vi "Get Selected Device info.vi"(0 "Boolean":bool, 5 "Selected Device":string, 9 "Virtual Devices Core Info":string[][](array[string]), 11 "error in (no error)":errorcluster) -> (4 "Virtual Device Variable List":string[](array[string]), 6 "Actual Device List":string[](array[string]), 8 ">Device Variables (Settable): Default val, Min, Max etc >":string[][](array[string]), 10 ">Selected Device>":string, 15 "error out":errorcluster)   [LabVIEW 2020]
uses:
  Shared/MySQL/Preset Query Enum.ctl
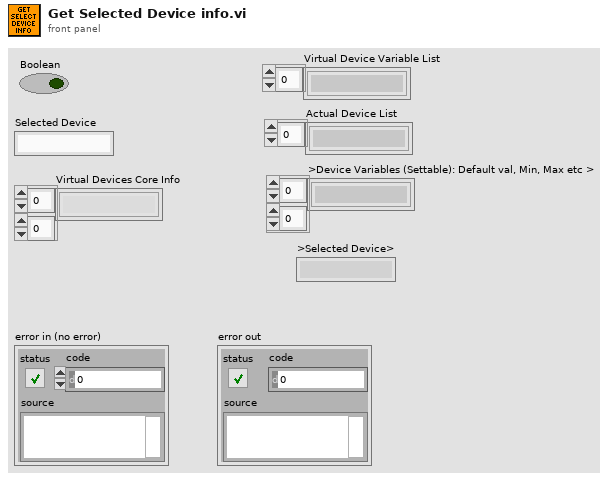
[diagram p1: front panel]
types:
  T1 = typedef "Preset Query Enum.ctl" = enum16{"Get Locations", "Get all IPs and MACs", "Get classes", "Get expt variables to set at scanstart for particular device", "Get expt devices and variables with start values", "Get expt devices and variables (with data to get)", "Get expt devices with data to get", "Get Expt devices and GUIs", "Get all devices basic properties", "Get Virtual Devices Core Info", "Get Expt names", "Get experiment basic properties", "Get experiment alarm variables", "Get MC Ports", "Get device network comm port", "Get devicetype lvclass path", "Get basic device properties", "Get Init Order", "Get all setable variables of a device", "Get device variable aliases", "Get force values of all settable variables", "Get all variables of a devicetype", "Get all variables of a device", "Get plotter details", "Get Saved Scans", "Get Scan Info", "GetGeneralGUIs", "Get expt for plotter", "Get plotter IDs from expt", "Get all devices", "Get all Virtual Devices", "Get all aliases", "Get variable and device info for Virtual Device", "GetItemLocatorIP", "Get IPs for GUIs", "Get DeviceType from Device", "GetLocalPortRange", "GetDevicePresetVariables", "Get Device Configuration", "GetAllPresetNames", "GetAllConfigurationNames", "GetPresetDeviceNames"}
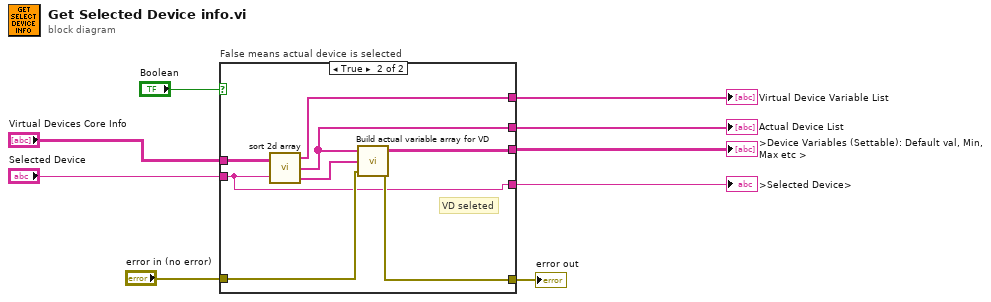
[diagram p0: block diagram]
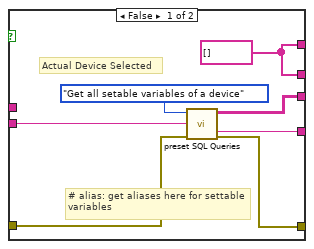
[diagram p2: hidden frame]
diagram:
  n1 = case "False means actual device is selected" shown="True" "Boolean" {
    tunnel: "Virtual Devices Core Info" -> [_ w23]
    tunnel: "Selected Device" -> [w12 w18]
    tunnel: [w14 w21] -> w9
    tunnel: "error in (no error)" -> [w13 w20]
    tunnel: [w11 w19] -> w3
    tunnel: [w12 w18] -> w8
    tunnel: [w10 w17] -> w5
    tunnel: [w10 w16] -> w6
    frame False {
      w10 = string[] [] ("array 4")
      # "# alias: get aliases here for settable\nvariables"
      # "Actual Device Selected"
      n2 = call "preset SQL Queries.vi"("error in (no error)"=w13, "Device/Devicetype name\n/Plotter.id/ScanName#"=w12, "Preset Query"=Preset_Query_Enum."Get all setable variables of a device") -> ("error out"=w11:errorcluster, "data"=w14:string[][])  [unwired: 6 in, 1 out]
    }
    frame True {
      # "VD seleted"
      n3 = call "sort 2d array.vi"("VD core Info"=w23, "Selected VD"=w18) -> ("Virtual Device Variable List"=w17:string[], "Actual Device List"=w16:string[], "Actual Variable List"=w22:string[])
      n4 = call "Build actual variable array for VD.vi"("error in"=w20, "Actual Variable List"=w22, "Actual Device List"=w16) -> ("error out"=w19:errorcluster, "appended array"=w21:string[][])  [unwired: 1 out]
    }
  }
  ">Device Variables (Settable): Default val, Min, Max etc >" <- w9
  ">Selected Device>" <- w8
  "Actual Device List" <- w6
  "Virtual Device Variable List" <- w5
  "error out" <- w3
